vi "Run.vi"(8 "error in (no error)":errorcluster, 9 "Audio Record Queue":refnum<queue>, 10 "Timing Source":string, 11 "Audio Output Queue":refnum<queue>) -> (0 "error out":errorcluster)   [LabVIEW 2020, in "Audio Engine.lvlib"]
doc: "The main audio processing loop.\n\n<b>Priority:</b> Above Normal\n<b>Execution System:</b> Standard"
uses:
  Audio Engine.lvlib
  Audio Output/Audio Output Queue Type.ctl
  <vilib>/Platform/TimedLoop/XDataNode/timing_clust.ctl
  <vilib>/Platform/TimedLoop/XDataNode/nitl_modes.ctl
  <vilib>/Platform/TimedLoop/XDataNode/wakeup.ctl
  Classes/Channel/EQ.vi
  Packed Libraries/Globals.lvlibp/Constants.vi
  Packed Libraries/Audio Processing.lvlibp/DBL To I16.vi
  <vilib>/platform/TimedLoop/XDataNode/XDataNode.xnode
  Classes/Deck/Deck.lvclass
  <vilib>/Platform/TimedLoop/XDataNode/XDNodeRunTimeDep.lvlib
  Audio Output/Audio Output.lvlib
  Packed Libraries/Globals.lvlibp
  Classes/Effect Unit/Effect Unit.lvclass
  Classes/Channel/Channel.lvclass
  Packed Libraries/Messaging.lvlibp
  Classes/Transport/Transport.lvclass
  Classes/Sample/Sample.lvclass
  Classes/Mixer/Mixer.lvclass
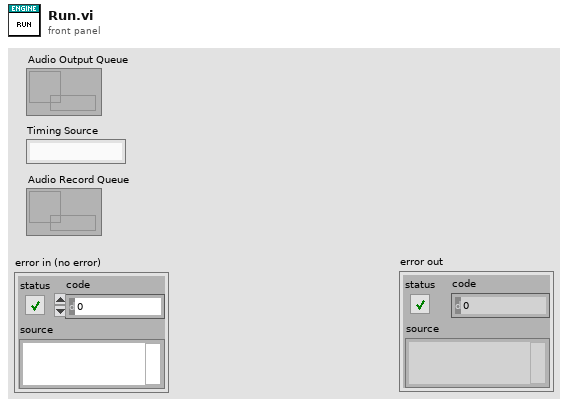
[diagram p1: front panel]
types:
  T1 = typedef "Audio Output.lvlib/Audio Output Queue Type.ctl" = cluster{"Master":waveform(i16)[], "Headphones":waveform(i16)[], "Start Time":dbl, "Record":bool}
  T2 = typedef "XDNodeRunTimeDep.lvlib/timing_clust.ctl" = cluster{"Expected End [f-1]":u64, "Actual End [f-1]":u64, "Finished Late? [f-1]":bool, "Expected End [i-1]":u64, "Actual End [i-1]":u64, "Finished Late? [i-1]":bool, "Expected Start [i]":u64, "Actual Start [i]":u64, "Expected Start [f]":u64, "Actual Start [f]":u64, "Source Name":string, "Structure Name":string, "Period":i64, "Deadline":i64, "Offset":i64, "Start":i64, "Priority":i32, "Timeout":i32, "Mode":T3, "Wakeup Reason":T4, "Error":errorcluster, "Source Type":string, "Secondary Source Type":string, "Global End Time":u64, "Global Start Time":u64, "Frame Duration":u64, "Iteration Duration":u64, "Assigned CPU":i32, "I/O Scan Engine Mode":u32}
  T3 = typedef "XDNodeRunTimeDep.lvlib/nitl_modes.ctl" = enum32{"No Change", "Process missed periods, maintain original phase", "Discard missed periods, maintain original phase", "Process missed periods, ignore original phase", "Discard missed periods, ignore original phase"}
  T4 = typedef "XDNodeRunTimeDep.lvlib/wakeup.ctl" = enum32{"Normal", "Aborted", "Asynchronous wakeup", "Timing source error", "Timed loop error", "Timeout"}
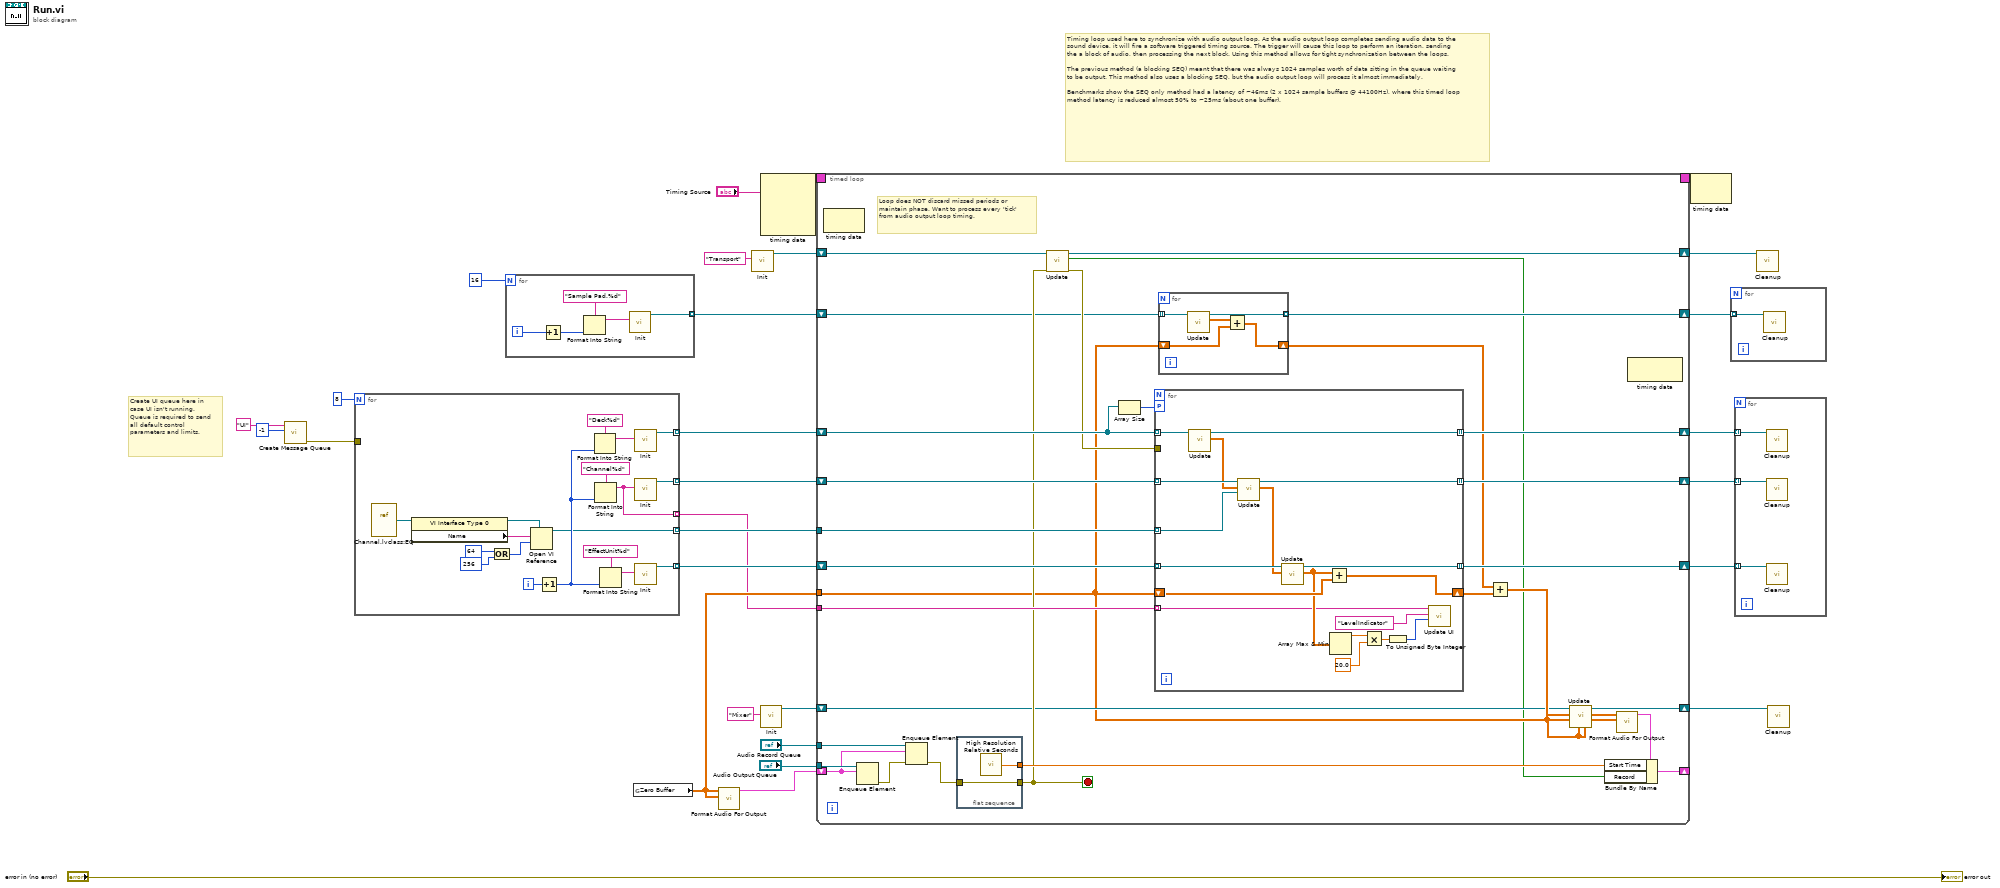
[diagram p0: block diagram]
diagram:
  # "Create UI queue here in case UI isn't running. Queue is required to send all default control parameters and limits."
  # "Timing loop used here to synchronize with audio output loop. As the audio output loop completes sending audio data to the sound device, it will fire a software triggered timing source. The trigger will cause this loop to perform an iteration, sending the a block of audio, then processing the next block. Using this method allows for tight synchronization between the loops.\n\nThe previous method (a blocking SEQ) meant that there was always 1024 samples worth of data sitting in the queue waiting to be output. This method also uses a blocking SEQ, but the audio output loop will process it almost immediately.\n\nBenchmarks show the SEQ only method had a latency of ~46ms (2 x 1024 sample buffers @ 44100Hz), where this timed loop method latency is reduced almost 50% to ~25ms (about one buffer)."
  n1 = call "Create Message Queue.vi"("Max Size (1000)"=-1, "Queue Name"="UI") -> ("error out"=w1:errorcluster)  [unwired: 8 in, 1 out]
  n2 = for {
    N: 8 -> [_]
    tunnel: [w40] -> w17 mode=indexing
    tunnel: [w39] -> w16 mode=indexing
    tunnel: [w38] -> w14 mode=indexing
    tunnel: [w31] -> w15 mode=indexing
    tunnel: [w30] -> w12 mode=indexing
    tunnel: w1 -> [_]
    i -> [w42]
    n3 = vi-ref "Channel.lvclass:EQ.vi"() -> (w37:refnum<vi>)
    n4 = property class="VI Interface Type 0"(reference=w37) -> (reference out=w35:refnum<vi>, "Name"=w36:string)  [unwired: 1 in, 1 out]
    n5 = Or(x=64 ("options"), y=256 ("options")) -> (x .or. y?=w32:i32)
    n6 = Open VI Reference(type specifier VI Refnum (for type only)=w35, vi path=w36, options=w32) -> (vi reference=w31:refnum<vi>)  [unwired: 3 in, 1 out]
    n7 = Increment(x=w42) -> (x+1=w41:i32)
    n8 = Format Into String(format string="Deck%d", w41) -> (resulting string=w44:string)  [unwired: 2 in, 1 out]
    n9 = Format Into String(format string="Channel%d", w41) -> (resulting string=w30:string)  [unwired: 2 in, 1 out]
    n10 = Format Into String(format string="EffectUnit%d", w41) -> (resulting string=w43:string)  [unwired: 2 in, 1 out]
    n11 = call "Init.vi"("ID"=w44) -> ("Deck out"=w40:refnum<class "Deck.lvclass">)  [unwired: 9 in, 1 out]
    n12 = call "Init.vi"("ID"=w30) -> ("Channel out"=w39:refnum<class "Channel.lvclass">)  [unwired: 9 in, 1 out]
    n13 = call "Init.vi"("ID"=w43) -> ("Effect Unit out"=w38:refnum<class "Effect Unit.lvclass">)  [unwired: 9 in, 1 out]
  }
  n14 = for {
    N: 16 -> [_]
    tunnel: [w49] -> w7 mode=indexing
    i -> [w51]
    n15 = Increment(x=w51) -> (x+1=w48:i32)
    n16 = Format Into String(format string="Sample Pad.%d", w48) -> (resulting string=w50:string)  [unwired: 2 in, 1 out]
    n17 = call "Init.vi"("ID"=w50) -> ("Deck out"=w49:refnum<class "Sample.lvclass">)  [unwired: 9 in, 1 out]
  }
  n18 = global read "Constants.vi" "Zero Buffer"() -> (w13:dbl[][])
  n19 = call "Format Audio For Output.vi"("Headphone Audio"=w13, "Master Audio"=w13) -> ("Audio Output"=w26:T1)  [unwired: 9 in]
  n20 = call "Init.vi"("ID"="Transport") -> ("Mixer out"=w10:refnum<class "Transport.lvclass">)  [unwired: 9 in, 1 out]
  n21 = node-c288("Timing Source") -> (w22:T2)  [unwired: 3 in]
  n22 = call "Init.vi"("ID"="Mixer") -> ("Mixer out"=w4:refnum<class "Mixer.lvclass">)  [unwired: 9 in, 1 out]
  n23 = timed-loop {
    shift-right: [w84] -> w27
    shift-left: w17 -> [w74]
    tunnel: "Audio Output Queue" -> [w83]
    timing: w22 -> [_]
    timing-out: [_] -> w21
    shift-right: [w80] -> _
    shift-left: w26 -> [w55]
    shift-right: [w76] -> w19
    shift-left: w14 -> [w77]
    shift-right: [w78] -> w20
    shift-left: w16 -> [w79]
    tunnel: w15 -> [w75]
    tunnel: w13 -> [w58]
    tunnel: w12 -> [w72]
    shift-right: [w68] -> w9
    shift-left: w10 -> [w71]
    shift-right: [w64] -> w6
    shift-left: w7 -> [w67]
    shift-right: [w61] -> w3
    shift-left: w4 -> [w62]
    tunnel: "Audio Record Queue" -> [w57]
    stop <- w70 stop-if-true
    # "Loop does NOT discard missed periods or maintain phase. Want to process every 'tick' from audio output loop timing."
    n24 = node-c288() -> ()  [unwired: 1 in, 1 out]
    n25 = Enqueue Element(queue=w83, element=w55) -> (error out=w54:errorcluster)  [unwired: 2 in, 2 out]
    n26 = Enqueue Element(queue=w57, element=w55, error in (no error)=w54) -> (error out=w53:errorcluster)  [unwired: 1 in, 2 out]
    n27 = flat-sequence {
      tunnel: [w91] -> w70
      tunnel: w53 -> [w91]
      tunnel: [w90] -> w82
      frame #0 {
        n28 = call <vilib>:"High Resolution Relative Seconds.vi"() -> ("relative seconds"=w90:dbl)
      }
    }
    n29 = call "Update.vi"("error in (no error)"=w70, "Mixer in"=w71) -> ("error out"=w69:errorcluster, "Record"=w56:bool, "Mixer out"=w68:refnum<class "Transport.lvclass">)  [unwired: 7 in]
    n30 = Array Size(array=w74) -> (size(s)=w73:i32)
    n31 = for {
      tunnel: w74 -> [w111] mode=indexing
      tunnel: [w110] -> w84 mode=indexing
      tunnel: w79 -> [w109] mode=indexing
      tunnel: [w108] -> w78 mode=indexing
      tunnel: w77 -> [w107] mode=indexing
      tunnel: [w106] -> w76 mode=indexing
      tunnel: w75 -> [w104] mode=indexing
      shift-right: [w101] -> w65
      shift-left: w58 -> [w102]
      workers-P: w73 -> [_]
      tunnel: w72 -> [w94] mode=indexing
      tunnel: w69 -> [_]
      n32 = call "Update.vi"("Deck in"=w111) -> ("Audio Block"=w105:dbl[][], "Deck out"=w110:refnum<class "Deck.lvclass">)  [unwired: 8 in, 1 out]
      n33 = call "Update.vi"("EQ VI Ref"=w104, "Audio Block In"=w105, "Channel in"=w109) -> ("Master Audio Block Out"=w103:dbl[][], "Channel out"=w108:refnum<class "Channel.lvclass">)  [unwired: 5 in, 2 out]
      n34 = call "Update.vi"("Audio Block In"=w103, "Effect Unit in"=w107) -> ("Audio Block Out"=w95:dbl[][], "Effect Unit out"=w106:refnum<class "Effect Unit.lvclass">)  [unwired: 7 in, 1 out]
      n35 = Add(x=w95, y=w102) -> (x+y=w101:dbl[][])
      n36 = Array Max & Min(array=w95) -> (max value=w98:dbl)  [unwired: 3 out]
      n37 = Multiply(x=w98, y=20.0) -> (x*y=w96:dbl)
      n38 = To Unsigned Byte Integer(number=w96) -> (unsigned 8bit integer=w100:u8)
      n39 = call "Update UI.vi"("Data"=w100, "Target"="LevelIndicator", "ID"=w94) -> ()  [unwired: 8 in, 1 out]
    }
    n40 = for {
      tunnel: w67 -> [w89] mode=indexing
      shift-right: [w86] -> w66
      shift-left: w58 -> [w87]
      tunnel: [w85] -> w64 mode=indexing
      n41 = call "Update.vi"("Deck in"=w89) -> ("Audio Block"=w88:dbl[][], "Deck out"=w85:refnum<class "Sample.lvclass">)  [unwired: 8 in, 1 out]
      n42 = Add(x=w88, y=w87) -> (x+y=w86:dbl[][])
    }
    n43 = Add(x=w66, y=w65) -> (x+y=w63:dbl[][])
    n44 = call "Update.vi"("Headphone Block 2"=w58, "Headphone Block 1"=w58, "Audio Block 2"=w58, "Audio Block 1"=w63, "Mixer in"=w62) -> ("Headphones Audio Block Out"=w59:dbl[][], "Master Audio Block Out"=w60:dbl[][], "Mixer out"=w61:refnum<class "Mixer.lvclass">)  [unwired: 3 in, 1 out]
    n45 = call "Format Audio For Output.vi"("Headphone Audio"=w59, "Master Audio"=w60) -> ("Audio Output"=w81:T1)  [unwired: 9 in]
    n46 = Bundle By Name(cluster=w81, "Start Time"=w82, "Record"=w56) -> (w80:T1)
    n47 = node-c288() -> ()  [unwired: 1 in, 1 out]
  }
  n48 = node-c288(w21) -> ()  [unwired: 1 out]
  n49 = for {
    tunnel: w6 -> [w112] mode=indexing
    n50 = call "Cleanup.vi"("Deck in"=w112) -> ()  [unwired: 9 in, 2 out]
  }
  n51 = for {
    tunnel: w27 -> [w115] mode=indexing
    tunnel: w20 -> [w114] mode=indexing
    tunnel: w19 -> [w113] mode=indexing
    n52 = call "Cleanup.vi"("Deck in"=w115) -> ()  [unwired: 9 in, 2 out]
    n53 = call "Cleanup.vi"("Channel in"=w114) -> ()  [unwired: 10 in, 1 out]
    n54 = call "Cleanup.vi"("Effect Unit in"=w113) -> ()  [unwired: 9 in, 2 out]
  }
  n55 = call "Cleanup.vi"("Mixer in"=w9) -> ()  [unwired: 10 in, 1 out]
  n56 = call "Cleanup.vi"("Mixer in"=w3) -> ()  [unwired: 10 in, 1 out]
  "error out" <- "error in (no error)"
